vi "1 Ch Digital Output.vi"(2 "Packet":u64, 4 "Digital Out Ch":refnum<k21>="Chassis1/Mod3/DO0") -> ()   [LabVIEW 2010]
uses:
  <vilib>/eio/EIONode/EIONode.xnode
  <vilib>/rvi/eio/nirviEIOImplementation/nirviEIOImplementation.xnode
  <vilib>/rvi/eio/common/nirviEmuClasses.ctl
  <vilib>/rvi/eio/common/nirviEmuTemplateMethod_noerrors.vi
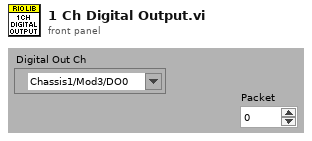
[diagram p1: front panel]
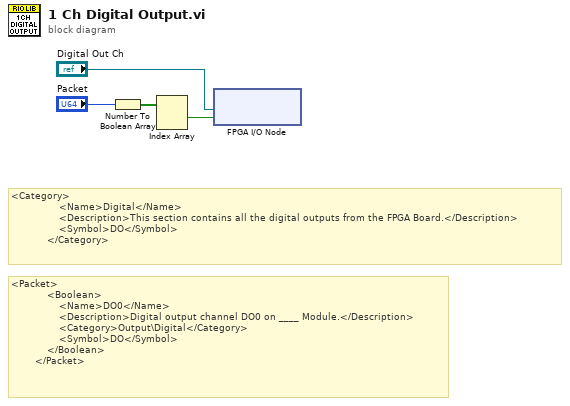
[diagram p0: block diagram]
diagram:
  # "<Category>\n                <Name>Digital</Name>\n                <Description>This section contains all the digital outputs from the FPGA Board.</Description>\n                <Symbol>DO</Symbol>\n            </Category>"
  # "<Packet>\n            <Boolean>\n                <Name>DO0</Name>\n                <Description>Digital output channel DO0 on ____ Module.</Description>\n                <Category>Output\\Digital</Category>\n                <Symbol>DO</Symbol>\n            </Boolean>\n        </Packet>"
  n1 = Number To Boolean Array(number="Packet") -> (Boolean array=w3:bool[])
  n2 = Index Array(array=w3) -> (element #1=w4:bool)  [unwired: 2 in, 1 out]
  n3 = xnode "FPGA I/O Node"("I/O Item"=w4, "FPGA I/O In"="Digital Out Ch") -> ()  [unwired: 1 out]
